vi "Robot Global Data.vi"() -> ()   [LabVIEW 2020]
doc: "This global VI can contain as many global variables as you need. To create a global variable, place a control on the panel, give it a good name. To read or write to it from a VI, drag the icon to the diagram of that VI. You can also drag from the project. Click on the node to change which global you access. You shouldn't have multiple locations writing to a global or it will cause a race-condition."
uses:
  <vilib>/Rock Robotics/WPI/Camera/WPI_CameraImageSize.ctl
  <vilib>/Rock Robotics/WPI/DriverStation/WPI_DriverStationRobotMode2.ctl
panel:
  in  "Auto Drive Time":dbl=3.0 format="%#_13g"
  in  "Auto Right Speed":dbl=0.5 format="%#_13g"
  in  "Auto Left Speed":dbl=0.5 format="%#_13g"
  in  "Auto Shoot Time":dbl=1.0 format="%#_13g"
  in  "Auto Shoot Set":dbl=-0.25 format="%#_13g"
  in  "Shooter Duration (s)":dbl=3.0 format="%#_13g"
  in  "Shooter Setpoint":dbl=0.8 format="%#_13g"
  in  "Intake Duration (s)":dbl=3.0 format="%#_13g"
  in  "Intake Setpoint":dbl=0.8 format="%#_13g"
  in  "Pivot Right Setpoint":dbl=0.4 format="%#_13g"
  in  "Pivot Left Setpoint":dbl=0.3 format="%#_13g"
  in  "Control Panel Duration (s)":dbl=3.0 format="%#_13g"
  in  "Control Panel Setpoint":dbl=0.8 format="%#_13g"
  in  "Climb Duration (s)":dbl=3.0 format="%#_13g"
  in  "Climb Setpoint":dbl=0.8 format="%#_13g"
  in  "Robot Mode":T1
  in  "image size":T2=enum."320x240"
  in  "Enable Vision":bool
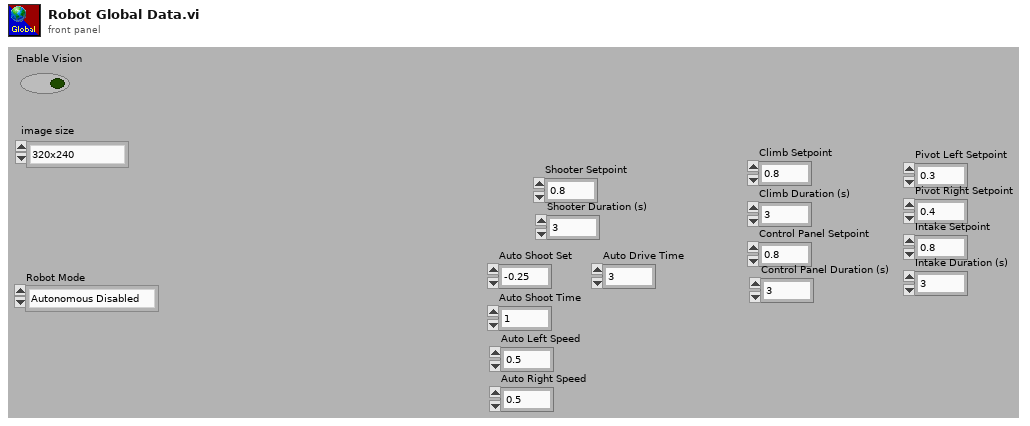
[diagram p1: front panel]
types:
  T1 = typedef "WPI_DriverStationRobotMode2.ctl" = enum16{"Autonomous Disabled", "Autonomous Enabled", "Teleop Disabled", "Teleop Enabled", "Disconnected", "Finish", "Test Disabled", "Test Enabled", "Emergency Stopped"}
  T2 = typedef "WPI_CameraImageSize.ctl" = enum16{"640x480", "320x240", "160x120", "Custom"}
diagram:
